vi "Read Tracking Data.vi"   [LabVIEW 2019]
uses:
  <vilib>/Rock Robotics/Network Tables/NT Read Number.vi
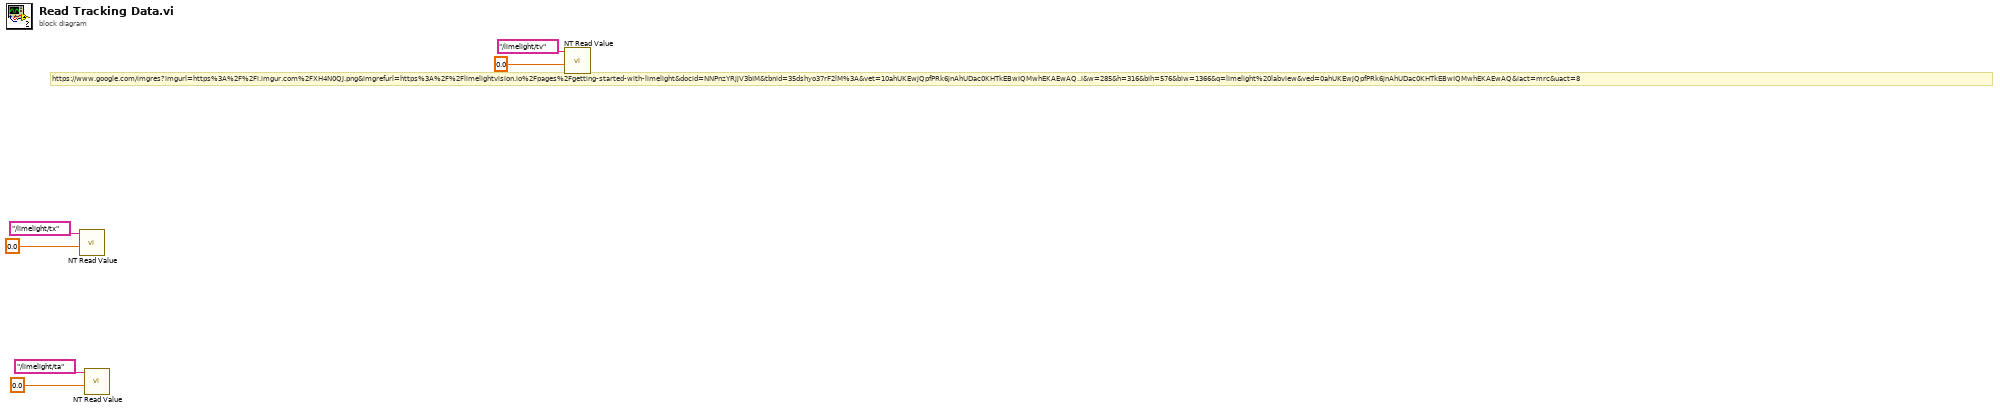
[diagram p0: block diagram]
diagram:
  # "https://www.google.com/imgres?imgurl=https%3A%2F%2Fi.imgur.com%2FXH4N0QJ.png&imgrefurl=https%3A%2F%2Flimelightvision.io%2Fpages%2Fgetting-started-with-limelight&docid=NNPnzYRjjV3bIM&tbnid=35dshyo37rF2lM%3A&vet=10ahUKEwjQpfPRk6jnAhUDac0KHTkEBwIQMwhEKAEwAQ..i&w=285&h=316&bih=576&biw=1366&q=limelight%20labview&ved=0ahUKEwjQpfPRk6jnAhUDac0KHTkEBwIQMwhEKAEwAQ&iact=mrc&uact=8"
  n1 = call-poly <vilib>:"NT Read Value.vi"("Default Value"=0.0, "Name"="/limelight/tx") -> ("Numeric"=w1:dbl)  [unwired: 8 in, 1 out]
  n2 = call-poly <vilib>:"NT Read Value.vi"("Default Value"=0.0, "Name"="/limelight/ta") -> ()  [unwired: 8 in, 2 out]
  n3 = call-poly <vilib>:"NT Read Value.vi"("Default Value"=0.0, "Name"="/limelight/tv") -> ()  [unwired: 8 in, 2 out]
